vi "MetaSaveCommandToPy.vi"(6 "MetaorMain":enum16{"Meta", "Main"}(ring), 8 "error in":errorcluster, 9 "Compiler Settings In":T1={"Python Path"=path "", "Main File"="makesequence.py", "Meta File"="makesequence.py", "Aux File"="makesequence.py", "Pre File"="metascript.txt"}, 11 "command":string) -> (0 "error out":errorcluster, 1 "Compiler Settings Out":T1={"Python Path"=path "", "Main File"="makesequence.py", "Meta File"="makesequence.py", "Aux File"="makesequence.py", "Pre File"="metascript.txt"})   [LabVIEW 2019]
uses:
  PulseCompiler/CompilerSettings.ctl
  controls/GlobalExp.vi
  Global.lvlib
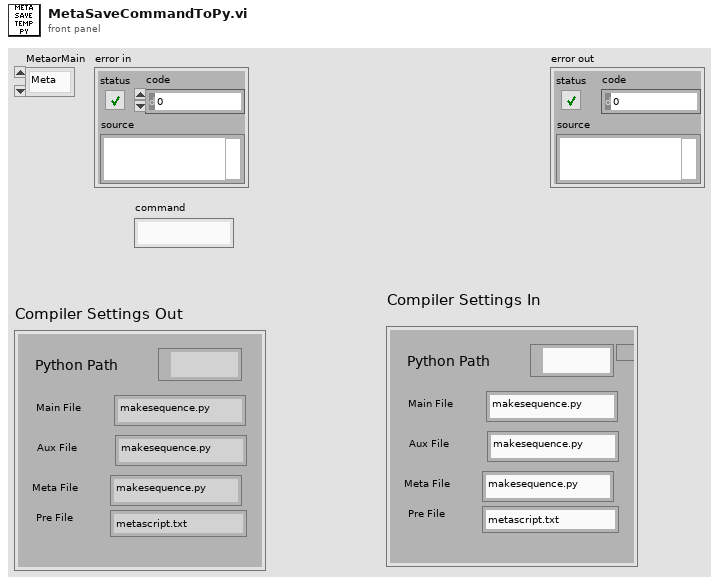
[diagram p1: front panel]
types:
  T1 = typedef "CompilerSettings.ctl" = cluster{"Python Path":path, "Main File":string, "Meta File":string, "Aux File":string, "Pre File":string}
  T2 = typedef "MasterExpControl.ctl" = cluster{"Main Steps":dbl, "Main Runs":dbl, "ExpStatus":enum16{"Innit", "Stop", "Idle", "MainRunning", "AuxRunning"}, "Main Current Step":dbl, "ExpNum":dbl, "NewData":bool, "date":string, "command":string, "Stop":bool, "Pause":bool, "Mathematica":string, "Main/Meta":bool, "UpdateMath":bool, "Camera":bool, "MetaExpOver":bool, "NextMetaExp":bool}
  T3 = enum16{"open", "replace", "create", "open or create", "replace or create", "replace or create with confirmation"}
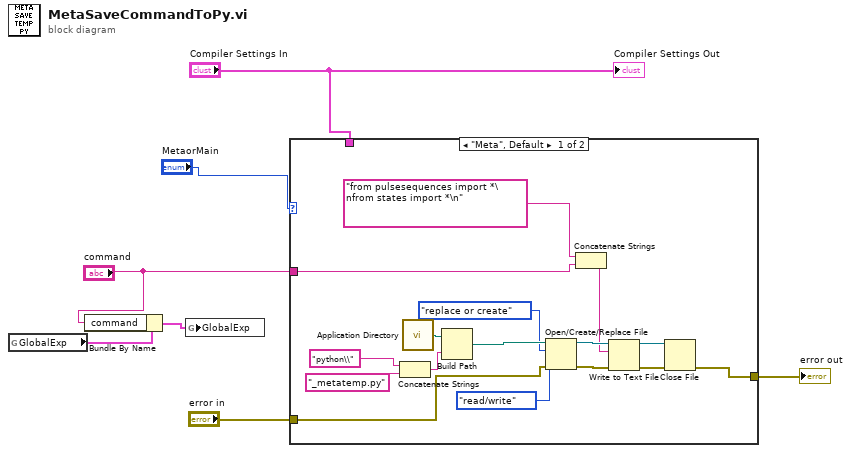
[diagram p0: block diagram]
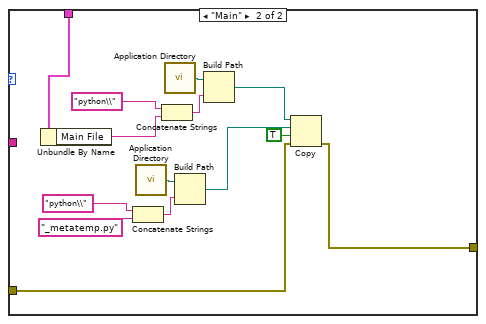
[diagram p2: hidden frame]
diagram:
  n1 = global read "GlobalExp.vi" "GlobalExp"() -> (w3:T2)
  n2 = Bundle By Name(cluster=w3, "command"="command") -> (w1:T2)
  n3 = global write "GlobalExp.vi" "GlobalExp"(w1) -> ()
  n4 = case shown="\"Meta\", Default" "MetaorMain" {
    tunnel: "Compiler Settings In" -> [_ w37]
    tunnel: "error in" -> [w10 w25]
    tunnel: [w9 w24] -> w4
    tunnel: "command" -> [w8 _]
    frame "Meta", Default {
      n5 = Concatenate Strings("python\\" ("name or relative path"), "_metatemp.py" ("string")) -> (w15:string)
      n6 = call <vilib>:"Application Directory.vi"() -> ("Application Directory"=w13:path)
      n7 = Build Path(base path=w13, name or relative path=w15) -> (appended path=w14:path)
      n8 = Open/Create/Replace File(file path (use dialog)=w14, error in=w10, operation (0:open)=T3."replace or create", access (0:read/write)=enum16{"read/write", "read-only", "write-only"}."read/write") -> (refnum out=w21:refnum<file>, error out=w22:errorcluster)  [unwired: 2 in, 1 out]
      n9 = Concatenate Strings("from pulsesequences import *\nfrom states import *\n", w8) -> (w11:string)
      n10 = Write to Text File(file (use dialog)=w21, text=w11, error in=w22) -> (refnum out=w19:refnum<file>, error out=w20:errorcluster)  [unwired: 1 in, 1 out]
      n11 = Close File(refnum=w19, error in=w20) -> (error out=w9:errorcluster)  [unwired: 1 out]
    }
    frame "Main" {
      n12 = Unbundle By Name(w37) -> ("Main File"=w27:string)
      n13 = Concatenate Strings("python\\" ("name or relative path"), "_metatemp.py" ("string")) -> (w35:string)
      n14 = call <vilib>:"Application Directory.vi"() -> ("Application Directory"=w36:path)
      n15 = Concatenate Strings("python\\" ("name or relative path"), w27) -> (w30:string)
      n16 = call <vilib>:"Application Directory.vi"() -> ("Application Directory"=w31:path)
      n17 = Build Path(base path=w36, name or relative path=w35) -> (appended path=w32:path)
      n18 = Build Path(base path=w31, name or relative path=w30) -> (appended path=w28:path)
      n19 = Copy(8:w25, 9:TRUE ("overwrite (F)"), 10:w32, 11:w28) -> (0:w24:errorcluster)  [unwired: 3 out]
    }
  }
  "error out" <- w4
  "Compiler Settings Out" <- "Compiler Settings In"
